vi "Ironbow Palette.vi"() -> (3 "Color Palette":cluster{"Red":u8, "Green":u8, "Blue":u8}[](array[cluster]))   [LabVIEW 2015]
panel:
  in  "String":string="0, 0, 0 \n0, 0, 36 \n0, 0, 51 \n0, 0, 66 \n0, 0, 81 \n2, 0, 90 \n4, 0, 99 \n7, 0, 106 \n11, 0, 115 \n14, 0, 119 \n20, 0, 123 \n27, 0, 128 \n33, 0, 133 \n41, 0, 137 \n48, 0, 140 \n55, 0, 143 \n61, 0, 146 \n66, 0, 149 \n72, 0, 150 \n78, 0, 151 \n84, 0, 152 \n91, 0, 153 \n97, 0, 155 \n104, 0, 155 \n110, 0, 156 \n115, 0, 157 \n122, 0, 157 \n128, 0, 157 \n134, 0, 157 \n139, 0, 157 \n146, 0, 156 \n152, 0, 155 \n157, 0, 155 \n162, 0, 155 \n167, 0, 154 \n171, 0, 153 \n175, 1, 152 \n178, 1, 151 \n182, 2, 149 \n185, 4, 149 \n188, 5, 147 \n191, 6, 146 \n193, 8, 144 \n195, 11, 142 \n198, 13, 139 \n201, 17, 135 \n203, 20, 132 \n206, 23, 127 \n208, 26, 121 \n210, 29, 116 \n212, 33, 111 \n214, 37, 103 \n217, 41, 97 \n219, 46, 89 \n221, 49, 78 \n223, 53, 66 \n224, 56, 54 \n226, 60, 42 \n228, 64, 30 \n229, 68, 25 \n231, 72, 20 \n232, 76, 16 \n234, 78, 12 \n235, 82, 10 \n236, 86, 8 \n237, 90, 7 \n238, 93, 5 \n239, 96, 4 \n240, 100, 3 \n241, 103, 3 \n241, 106, 2 \n242, 109, 1 \n243, 113, 1 \n244, 116, 0 \n244, 120, 0 \n245, 125, 0 \n246, 129, 0 \n247, 133, 0 \n248, 136, 0 \n248, 139, 0 \n249, 142, 0 \n249, 145, 0 \n250, 149, 0 \n251, 154, 0 \n252, 159, 0 \n253, 163, 0 \n253, 168, 0 \n253, 172, 0 \n254, 176, 0 \n254, 179, 0 \n254, 184, 0 \n254, 187, 0 \n254, 191, 0 \n254, 195, 0 \n254, 199, 0 \n254, 202, 1 \n254, 205, 2 \n254, 208, 5 \n254, 212, 9 \n254, 216, 12 \n255, 219, 15 \n255, 221, 23 \n255, 224, 32 \n255, 227, 39 \n255, 229, 50 \n255, 232, 63 \n255, 235, 75 \n255, 238, 88 \n255, 239, 102 \n255, 241, 116 \n255, 242, 134 \n255, 244, 149 \n255, 245, 164 \n255, 247, 179 \n255, 248, 192 \n255, 249, 203 \n255, 251, 216 \n255, 253, 228 \n255, 254, 239 \n255, 255, 249"
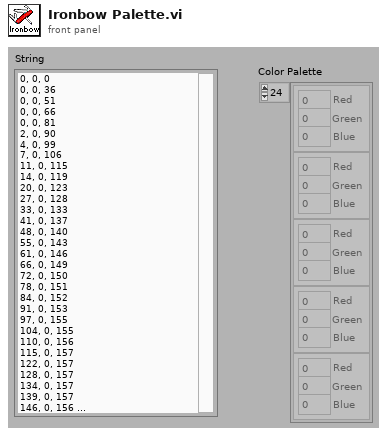
[diagram p1: front panel]
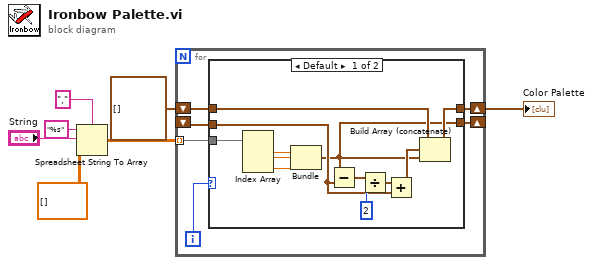
[diagram p0: block diagram]
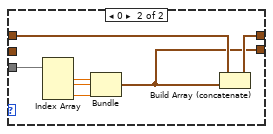
[diagram p2: hidden frame]
diagram:
  n1 = Spreadsheet String To Array(delimiter (Tab)=",", format string="%s", spreadsheet string="String", array type (2D Dbl)=dbl[][] []) -> (array=w3:dbl[][])
  n2 = for {
    tunnel: w3 -> [w13] mode=indexing
    shift-right: [w11] -> w2
    shift-left: cluster{dbl, dbl, dbl}[] [] -> [w12]
    shift-right: [w9] -> _
    shift-left: _ -> [w8]
    i -> [w10]
    n3 = case shown="Default" w10 {
      tunnel: w13 -> [w25 w32]
      tunnel: w12 -> [w21 w28]
      tunnel: [w20 w27] -> w11
      tunnel: [w14 w26] -> w9
      tunnel: w8 -> [w16 _]
      frame Default {
        n4 = Index Array(array=w25) -> (element #1=w24:dbl, element #2=w22:dbl, element #3=w23:dbl)  [unwired: 3 in]
        n5 = Bundle(w24, w22, w23) -> (w14:cluster{dbl, dbl, dbl})  [unwired: 1 in]
        n6 = Subtract(x=w14, y=w16) -> (x-y=w19:cluster{dbl, dbl, dbl})
        n7 = Divide(x=w19, y=2) -> (x/y=w17:cluster{dbl, dbl, dbl})
        n8 = Add(x=w17, y=w16) -> (x+y=w15:cluster{dbl, dbl, dbl})
        n9 = Build Array (concatenate)(w21, w15, w14) -> (w20:cluster{dbl, dbl, dbl}[])
      }
      frame 0 {
        n10 = Index Array(array=w32) -> (element #1=w31:dbl, element #2=w29:dbl, element #3=w30:dbl)  [unwired: 3 in]
        n11 = Bundle(w31, w29, w30) -> (w26:cluster{dbl, dbl, dbl})  [unwired: 1 in]
        n12 = Build Array (concatenate)(w28, w26) -> (w27:cluster{dbl, dbl, dbl}[])
      }
    }
  }
  "Color Palette" <- w2
